vi "Process_ROI_Image.vi"(4 "Dllindex":i32, 6 "CreatDllImage":bool, 8 "error in (no error)":errorcluster, 9 "ForCalCalculaton In":T1, 10 "ROI Entry":T2={"vROIName"="", "vROIContour"={"Contour Type"=0, "ROI Type"=0, "Points"=[]}, "ProcessSetting"=[], "Analysis_Setting"={"PreProcess"=enum."*Algorithm*", "Parameter"=""}}, 11 "ImageIn":T1(plugin-control)) -> (0 "error out":errorcluster, 1 "ForCalCalculaton Out":T1, 3 "ExtractedProcessedImage":T1(plugin-control))   [LabVIEW 2019]
uses:
  <vilib>/vision/NI_Vision_Development_Module.lvlib
  DLL/[Global] OperatorsImageTemplate2.vi
  DLL/[Global] ExtractedProcessImage.vi
  Controls/Parameter.ctl
  Process/Controls/Process_Setting.ctl
  Analysis/Controls/Analysis_Setting.ctl
  Controls/Vision_DataEntry.ctl
  <vilib>/vision/Image Controls.llb/IMAQ Image.ctl
  Ctrl/VisionProcessName.ctl
panel:
  out "Image Type":T7 items=["Grayscale (U8)", "Grayscale (I16)", "Grayscale (SGL)", "Complex (CSG)", "RGB (U32)", "HSL (U32)", "RGB (U64)", "Grayscale (U16)"]
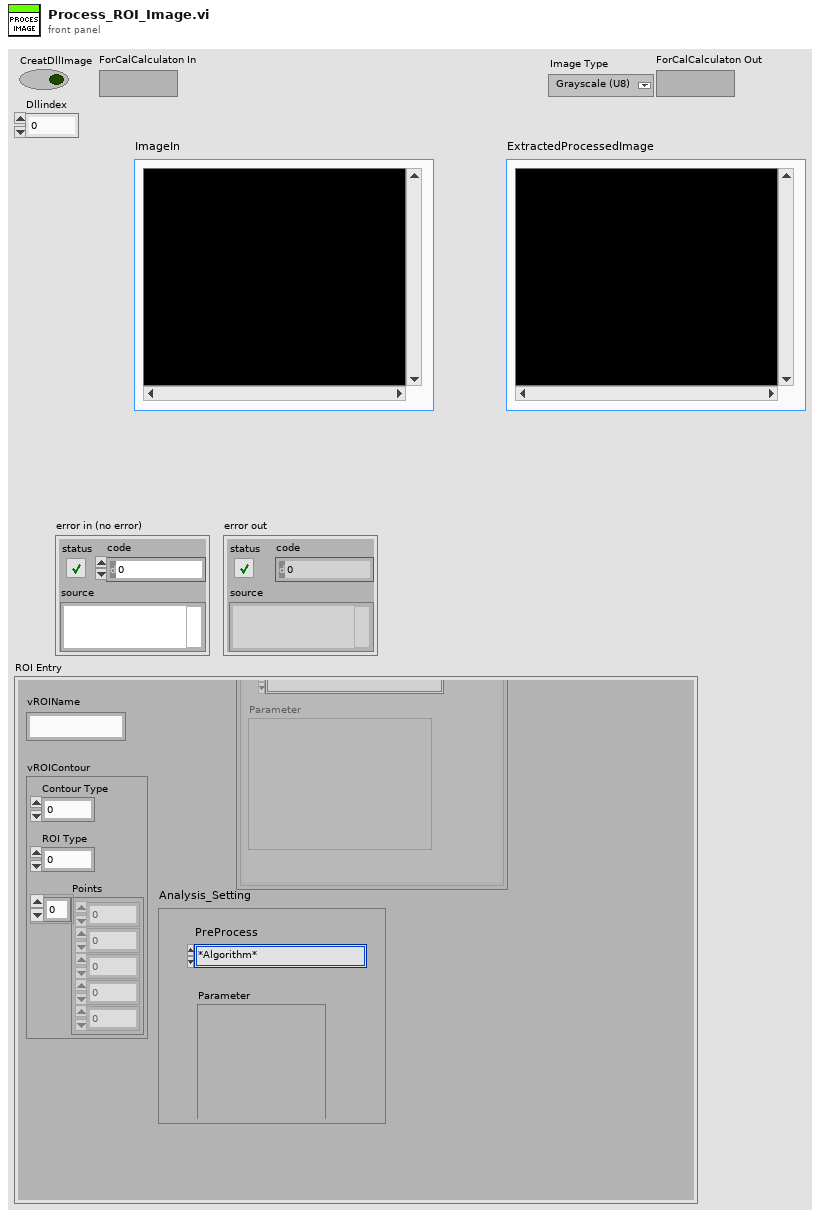
[diagram p1: front panel]
types:
  T1 = typedef "IMAQ Image.ctl" = refnum<image>
  T2 = typedef "Vision_DataEntry.ctl" = cluster{"vROIName":string, "vROIContour":cluster{"Contour Type":u32, "ROI Type":u32, "Points":i32[]}, "ProcessSetting":T3[], "Analysis_Setting":T5}
  T3 = typedef "Process_Setting.ctl" = cluster{"Enum_PreProcess":T4, "Parameter":string}
  T4 = typedef "VisionProcessName.ctl" = enum16{"*CamParameter*", "CamAttributes", "*Preprocess*", "CG_Brightness", "C_Plane Extraction", "C_Threshold", "G_Lookup Table", "G_Threshold"}
  T5 = typedef "Analysis_Setting.ctl" = cluster{"PreProcess":T6, "Parameter":string}
  T6 = typedef "VisionProcessName.ctl" = enum16{"*CamParameter*", "CamAttributes", "*Preprocess*", "CG_Brightness", "C_Plane Extraction", "C_Threshold", "G_Lookup Table", "G_Threshold", "B_Image Inversion", "*Algorithm*", "CG_Histogram", "C_Color Matching", "C_Color Pattern Matching", "G_PatternMatch", "CG_Find Straight Edge", "CG_Adv. Find Straight Edge", "CG_Find Circular Edge", "G_Max Clamp", "G_Clamp (Rake)", "G_Pattern Matching"}
  T7 = typedef "Image Type" = u32
  T8 = typedef "Parameter.ctl" = enum16{"Initialize", "Write", "Read", "WriteAll", "Save", "Load"}
  T9 = cluster{"Contour Type":u32, "ROI Type":u32, "Points":i32[]}
  T10 = typedef "ParameterData.ctl" = cluster{"Rotate Angle":dbl, "Rotate?":bool, "Calibration File Path":string, "Cal?":bool}
  T11 = cluster{"Contour Type":u32, "ROI Type":u32, "Points":i32[]}[]
  T12 = cluster{"Points":i32[], cluster{"Contour Type":u32, "ROI Type":u32, "Points":i32[]}[]}
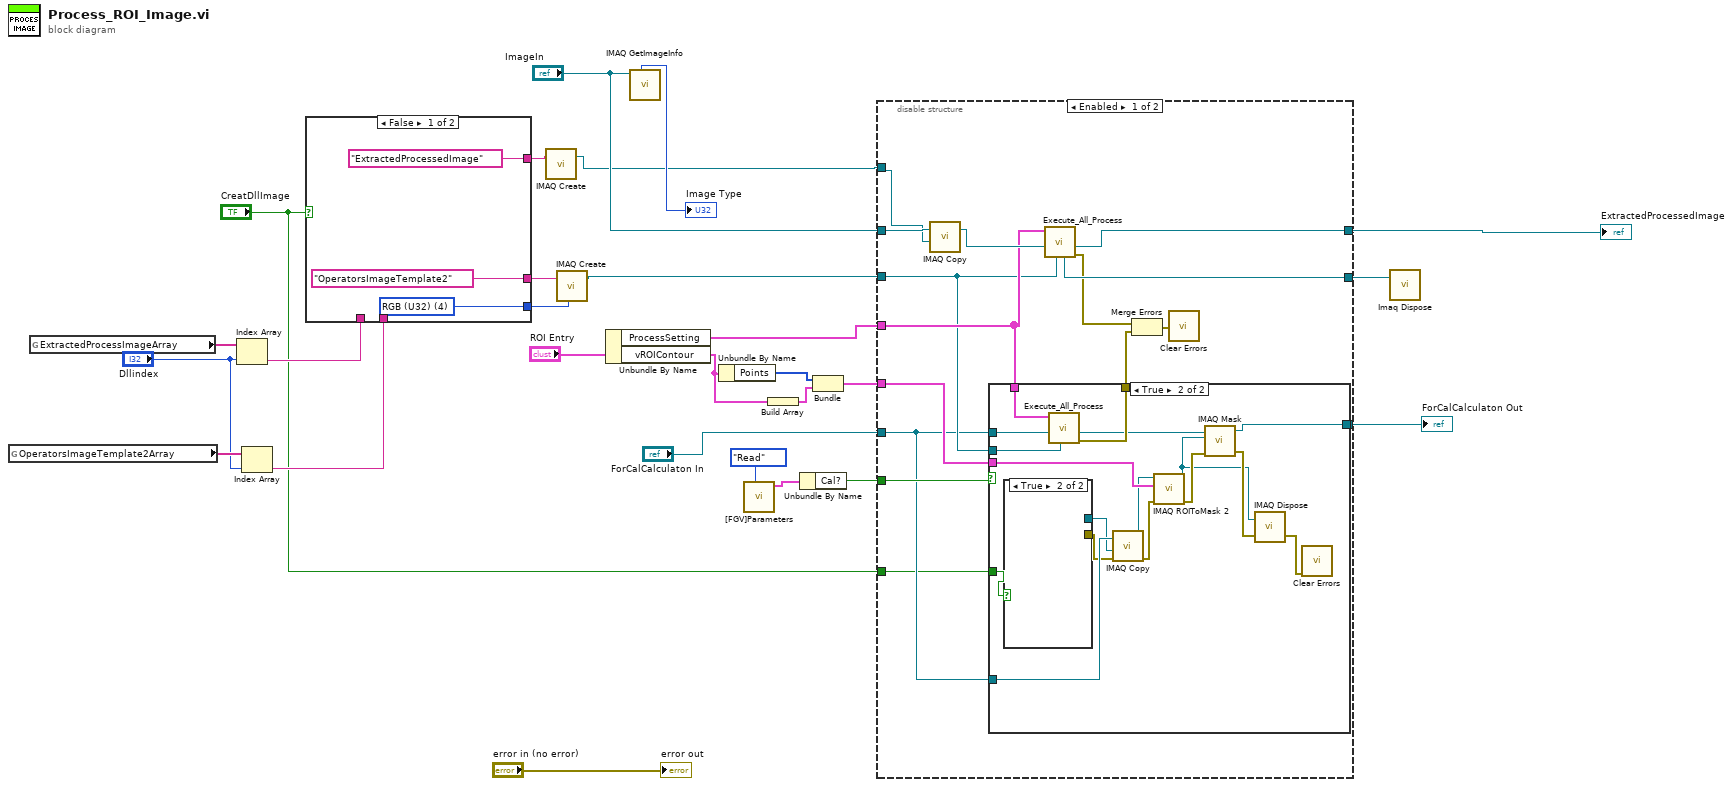
[diagram p0: block diagram]
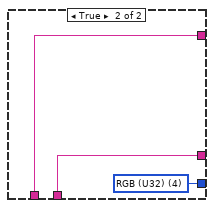
[diagram p2: hidden frame]
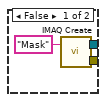
[diagram p4: hidden frame]
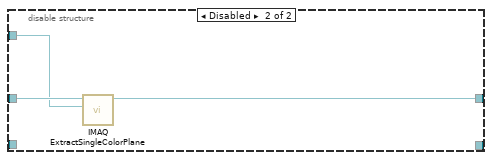
[diagram p5: hidden frame]
diagram:
  n1 = global read "[Global] OperatorsImageTemplate2.vi" "OperatorsImageTemplate2Array"() -> (w20:string[])
  n2 = global read "[Global] ExtractedProcessImage.vi" "ExtractedProcessImageArray"() -> (w21:string[])
  n3 = Index Array(array=w21, index="Dllindex") -> (element=w13:string)
  n4 = Index Array(array=w20, index="Dllindex") -> (element=w12:string)
  n5 = case shown="False" "CreatDllImage" {
    tunnel: ["ExtractedProcessedImage" ("Image Name") w33] -> w18
    tunnel: ["OperatorsImageTemplate2" ("Image Name") w31] -> w17
    tunnel: [w28 w32] -> w16
    tunnel: w13 -> [_ w33]
    tunnel: w12 -> [_ w31]
    frame False {
      w28 = T7 4 items=["Grayscale (U8)", "Grayscale (I16)", "Grayscale (SGL)", "Complex (CSG)", "RGB (U32)", "HSL (U32)", "RGB (U64)", "Grayscale (U16)"] ("Image Type")
    }
    frame True {
      w32 = T7 4 items=["Grayscale (U8)", "Grayscale (I16)", "Grayscale (SGL)", "Complex (CSG)", "RGB (U32)", "HSL (U32)", "RGB (U64)", "Grayscale (U16)"] ("Image Type")
    }
  }
  n6 = call "IMAQ Create"("Image Name"=w18) -> ("New Image"=w15:T1)  [unwired: 4 in, 1 out]
  n7 = call "IMAQ Create"("Image Name"=w17, "Image Type"=w16) -> ("New Image"=w14:T1)  [unwired: 2 in, 2 out]
  n8 = Unbundle By Name("ROI Entry") -> ("ProcessSetting"=w24:T3[], "vROIContour"=w4:T9)
  n9 = call "IMAQ GetImageInfo"("Image"="ImageIn") -> ("Image Type"=→"Image Type":T7)  [unwired: 3 in, 7 out]
  n10 = Unbundle By Name(w4) -> ("Points"=w5:i32[])
  n11 = call "[FGV]Parameters.vi"("Parameter"=Parameter."Read") -> ("ParameterData Out"=w7:T10)  [unwired: 9 in, 1 out]
  n12 = Build Array(w4) -> (w3:T11)
  n13 = Unbundle By Name(w7) -> ("Cal?"=w6:bool)
  n14 = Bundle("Points"=w5, w3) -> (w2:T12)  [unwired: 1 in]
  n15 = disable-structure shown="Enabled" {
    disable-tunnel: "ImageIn" -> [w48 w72]
    disable-tunnel: [w45 w70] -> w26
    disable-tunnel: w15 -> [w47 w71]
    disable-tunnel: w24 -> [w43 _]
    disable-tunnel: w14 -> [w42 _]
    disable-tunnel: [w44 _] -> w23
    disable-tunnel: "ForCalCalculaton In" -> [w35 _]
    disable-tunnel: [w38 _] -> w9
    disable-tunnel: w6 -> [w37 _]
    disable-tunnel: w2 -> [w36 _]
    disable-tunnel: "CreatDllImage" -> [w34 _]
    frame Enabled {
      n16 = call "IMAQ Copy"("Image Dst"=w47, "Image Src"=w48) -> ("Image Dst Out"=w46:T1)  [unwired: 4 in, 1 out]
      n17 = case shown="True" w37 {
        tunnel: w35 -> [w49 w66]
        tunnel: w43 -> [_ w65]
        tunnel: w42 -> [_ w64]
        tunnel: [_ w63] -> w40
        tunnel: [w49 w57] -> w38
        tunnel: w36 -> [_ w62]
        tunnel: w35 -> [_ w61]
        tunnel: w34 -> [_ w52]
        frame False {
        }
        frame True {
          n18 = case shown="True" w52 {
            tunnel: [w68 _] -> w60
            tunnel: [w67 _] -> w50
            frame False {
              n19 = call "IMAQ Create"("Image Name"="Mask") -> ("New Image"=w68:T1, "error out"=w67:errorcluster)  [unwired: 3 in, 1 out]
            }
            frame True {
            }
          }
          n20 = call "Execute_All_Process.vi"("OperatorImage In"=w64, "ImageIn"=w66, "ProcessSettingIn"=w65) -> ("error out"=w63:errorcluster, "Image Out"=w58:T1)  [unwired: 3 in, 4 out]
          n21 = call "IMAQ Copy"("error in (no error)"=w50, "Image Dst"=w60, "Image Src"=w61) -> ("error out"=w56:errorcluster, "Image Dst Out"=w59:T1)  [unwired: 3 in]
          n22 = call "IMAQ ROIToMask 2"("error in (no error)"=w56, "ROI Descriptor"=w62, "Image"=w59) -> ("error out"=w55:errorcluster, "Image Out"=w53:T1)  [unwired: 6 in, 1 out]
          n23 = call "IMAQ Mask"("error in (no error)"=w55, "Image Mask"=w53, "Image Src"=w58) -> ("error out"=w54:errorcluster, "Image Dst Out"=w57:T1)  [unwired: 2 in]
          n24 = call "IMAQ Dispose"("Image"=w53, "error in (no error)"=w54) -> ("error out"=w51:errorcluster)  [unwired: 4 in]
          n25 = call <vilib>:"Clear Errors.vi"("error in (no error)"=w51) -> ()  [unwired: 5 in, 2 out]
        }
      }
      n26 = call "Execute_All_Process.vi"("OperatorImage In"=w42, "ImageIn"=w46, "ProcessSettingIn"=w43) -> ("error out"=w41:errorcluster, "Image Out"=w45:T1, "OperatorImage Out"=w44:T1)  [unwired: 3 in, 3 out]
      n27 = Merge Errors(w41, w40) -> (w39:errorcluster)
      n28 = call <vilib>:"Clear Errors.vi"("error in (no error)"=w39) -> ()  [unwired: 5 in, 2 out]
    }
    frame Disabled {
      n29 = call "IMAQ ExtractSingleColorPlane"("Image Dst"=w71, "Image Src"=w72) -> ("Image Dst Out"=w70:T1)  [unwired: 8 in, 1 out]
    }
  }
  "ExtractedProcessedImage" <- w26
  "ForCalCalculaton Out" <- w9
  n30 = call "Imaq Dispose"("Image"=w23) -> ()  [unwired: 5 in, 1 out]
  "error out" <- "error in (no error)"
